vi "LCOS Exit Global.vi"() -> ()   [LabVIEW 2011]
panel:
  in  "Exit":bool
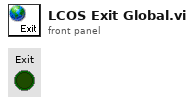
[diagram p1: front panel]
diagram:
